vi "CreateWyPtDict.vi"(8 "error in (no error)":errorcluster, 10 "Waypoint Dictionary ConfigFile":path=path "C:/Projects/BRS-Dev/BRS Information/Waypoint Dictionary Configuration File.xml") -> (0 "error out":errorcluster, 2 "WyPt Dict":T1)   [LabVIEW 2020, in "WyPtDict.lvlib"]
doc: "Developed by Kevin Thompson\nkevin@thompsonengineering.net\n\nCopyright 2021\nThompson Engineering, LLC"
uses:
  WyPtDict.lvlib
  support/MC and Robo Handshake.ctl
  RoboWaypointDict Node--cluster.ctl
  WyPtFullNode--cluster.ctl
  StockerExpansionModuleID--enum.ctl
  <vilib>/TELLC/Dynamic CVT API/TD Dynamic CVT DVR--ref.ctl
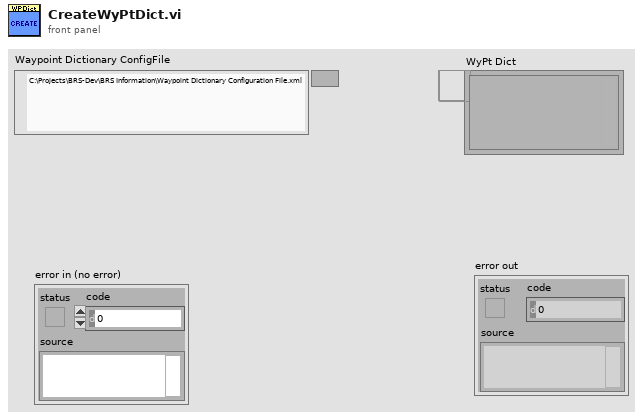
[diagram p1: front panel]
types:
  T1 = typedef "TD Dynamic CVT DVR--ref.ctl" = refnum<data-value>
  T2 = typedef "WyPtDict.lvlib/WyPtFullNode--cluster.ctl" = cluster{"WPArray":string[], "RoboWaypointDict Node":T3}
  T3 = typedef "WyPtDict.lvlib/RoboWaypointDict Node--cluster.ctl" = cluster{"MC and Robo Handshake":T4, "Idx":i32, "Cmd Number":string, "Waypoint List":string, "Description":string, "ExpMod ID":T5}
  T4 = typedef "MC and Robo Handshake.ctl" = enum16{"None", "Move and Pick Nikon Ret LP(1100)", "Nikon Barcode1 Scanning Started(1101)", "Nikon Barcode1 Scan Abort(1102)", "Nikon Barcode1 Scan Success Proc to Barcode 2 Pos(1103)", "Nikon Barcode 2 Scanning Started(1104)", "Nikon Barcode 2 Scan Abort(1105) ", "Nikon Barcode 2 Success(1106)", "Move and Pick POZZ Ret LP(1300)", "POZZ Barcode Scan Started(1301)", "POZZ Barcode Not Found(1302)", "POZZ Barcode Scan Succ(1303)", "POZZ Mov to Side 2 Bar 2(1310)", "POZZ Mov to Side 4 Bar 1(1311)", "POZZ Mov to Side 4 Bar 2(1312)", "POZZ Mov to Side 1 Bar 1(1313)", "POZZ Mov to Side 1 Bar 2(1314)", "POZZ Mov to Side 3 Bar 1(1315)", "POZZ Mov to Side 3 Bar 2(1316)", "POZZ Mov to Edge 3 Nik 2(1317)", "POZZ Mov to Edge 4 ASML(1318)", "POZZ Mov to Edge 4 Nik 1(1319)", "POZZ Mov to Edge 4 Nik 2(1320)", "Move to ASML LP and Pick Ret(2000)", "ASML1 Barcode Scan Started(2001)", "ASML1 Barcode Not Found(2002)", "ASML1 Barcode Scan Succ(2003)", "Start Load Seq for Nikon LP(3000)", "Start Load Seq for POZZ LP(3200)", "Start Load Seq for ASML LP(3400)", "Start Align End Grip Place Func(4000)", "Start Align End grip Pick Func(4001)", "Start Align Center Grip Place Func(4002)", "Start Align Center grip Pick Func(4003)", "Start Move from home to Cleaner(5000)", "Start Move to Final Cleaner Loc(5001)", "Start Move from Cleaner loc to home(5002)", "Start Move from home to PDS for Inspect(6000) ", "PDS Inspect Finished(6001)", "PDS EMO Recovery(6002)", "Store in Stocker(7001)", "Store in Expansion Stocker(7402)", "Retrive from Center Stocker(8001)", "Retrive Mov to Nikon BC1 Scan Pos(8002)", "Retrive Nikon BC1not found(8003)", "Retrive Nikon BC1 Scan Succ(8004)", "Retrive Nikon BC2 not found(8005)", "Retrive Nikon BC2 scan Succ(8006)", "Retrive Mov to Edge 1 ASML(8202) ", "Retrive Mov to Edge 1 Nikon 1(8203)", "Retrive Mov to Edge 1 Nikon 2(8204)", "Retrive Mov to Edge 2 ASML(8205)", "Retrive Mov to Edge 2 Nikon 1(8206)", "Retrive Mov to Edge 2 Nikon 2(8207)", "Retrive Mov to Edge 3 ASML (8208)", "Retrive Mov to Edge 3 Nikon 1(8209)", "Retrive Mov to Edge 3 Nikon 2(8210)", "Retrive Mov to Edge 4 ASML (8211)", "Retrive Mov to Edge 4 Nikon 1 (8212)", "Retrive Mov to Edge 4 Nikon 2 (8213)", "Retrive BC Scan Abort (8214)", "Retrive BC Scan Successful (8215)", "Retrive Mov to ASML BC scan Pos (8402) ", "Retrive ASML BC not found(8403)", "Retrive ASML BC Scan Succ(8404)", "Expansion Retrive Seq (8602)", "Cen Stocker move from home to Transit Nest(9000)", "Cen Stocker move from Transit Nest to home(9200)", "Exp Stocker move from home to Transit Nest(9400)", "Exp Stocker move from Transit Nest to home(9600)", "Move to R1 Home (1000)", "Move to R2 Home (1111)", "Store Left Stocker (7401)", "Retrieve Left Stocker (8601)", "EMO Recovery Center (1002)", "EMO Recovery Right (1003)", "Center Robo Status (8888)", "Right Robo Status (8889)"}
  T5 = typedef "WyPtDict.lvlib/StockerExpansionModuleID--enum.ctl" = enum16{"None", "Main", "Exp1", "Exp2", "Exp3", "Exp4", "Exp5"}
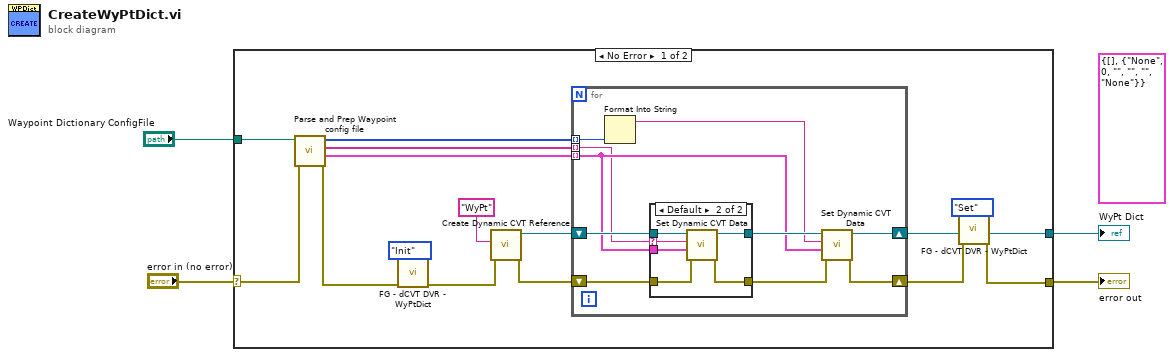
[diagram p0: block diagram]
diagram:
  (unwired) T2 {"WPArray"=[], "RoboWaypointDict Node"={"MC and Robo Handshake"=enum."None", "Idx"=0, "Cmd Number"="", "Waypoint List"="", "Description"="", "ExpMod ID"=enum."None"}} ("WyPtFullNode")
  n1 = case shown="No Error" "error in (no error)" {
    selector: "error in (no error)" -> [w10 w39]
    tunnel: [w13 _] -> w4
    tunnel: [w11 w39] -> w3
    tunnel: "Waypoint Dictionary ConfigFile" -> [w9 _]
    frame No Error {
      n2 = call "Parse and Prep Waypoint config file.vi"("error in (no error)"=w10, "Waypoint Dictionary ConfigFile"=w9) -> ("error out"=w5:errorcluster, "WyPtFullNode[]"=w6:T2[], "CmdNumber[]"=w7:string[], "Handshake[]"=w8:T4[])  [unwired: 5 in, 1 out]
      n3 = call "FG - dCVT DVR - WyPtDict.vi"("error in (no error)"=w5, "Action (Get)"=enum16{"Init", "Get", "Set"}."Init") -> ("error out"=w17:errorcluster)  [unwired: 7 in, 1 out]
      n4 = call <vilib>:"Create Dynamic CVT Reference.vi"("error in (no error)"=w17, "DictName"="WyPt") -> ("error out"=w19:errorcluster, "dCVT DVR out"=w18:T1)  [unwired: 8 in]
      n5 = for {
        shift-right: [w25] -> w12
        shift-left: w19 -> [w29]
        shift-right: [w24] -> w15
        shift-left: w18 -> [w30]
        tunnel: w8 -> [w28] mode=indexing
        tunnel: w7 -> [w21] mode=indexing
        tunnel: w6 -> [w22] mode=indexing
        n6 = Format Into String(w28) -> (resulting string=w23:string)  [unwired: 3 in, 1 out]
        n7 = case shown="Default" w21 {
          selector: w21 -> [_ w33]
          tunnel: w30 -> [w32 w38]
          tunnel: w29 -> [w31 w37]
          tunnel: [w32 w36] -> w27
          tunnel: [w31 w35] -> w26
          tunnel: w22 -> [_ w34]
          frame "" {
          }
          frame Default {
            n8 = call <vilib>:"Set Dynamic CVT Data.vi"("error in (no error)"=w37, "value"=w34, "DataName"=w33, "dCVT DVR"=w38) -> ("error out"=w35:errorcluster, "dCVT DVR out"=w36:T1)  [unwired: 5 in, 1 out]
          }
        }
        n9 = call <vilib>:"Set Dynamic CVT Data.vi"("error in (no error)"=w26, "value"=w22, "DataName"=w23, "dCVT DVR"=w27) -> ("error out"=w25:errorcluster, "dCVT DVR out"=w24:T1)  [unwired: 5 in, 1 out]
      }
      n10 = call "FG - dCVT DVR - WyPtDict.vi"("dCVT WyPt"=w15, "error in (no error)"=w12, "Action (Get)"=enum16{"Init", "Get", "Set"}."Set") -> ("dCVT WyPt out"=w13:T1, "error out"=w11:errorcluster)  [unwired: 6 in]
    }
    frame Error {
    }
  }
  "WyPt Dict" <- w4
  "error out" <- w3
